vi "mux10_1(x6)_encode.vi"(8 "error in (no error)":errorcluster, 10 "mux10_1(x6)_encode":T1(ring), 11 "Mem_mapping in":u16[](array[numeric])) -> (0 "error out":errorcluster, 3 "MemMapping Out":u16[](array[numeric]))   [LabVIEW 2018, in "MB Relay.lvlib"]
uses:
  MB Relay.lvlib
panel:
  out "mux1_10(x6)":u16[](array[numeric])
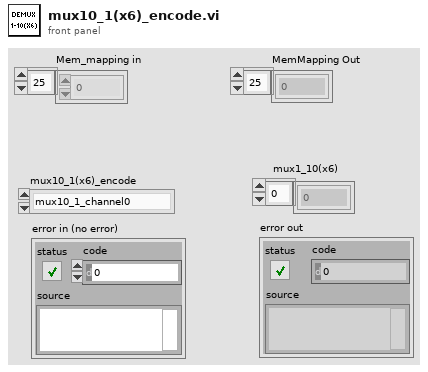
[diagram p1: front panel]
types:
  T1 = enum16{"mux10_1_channel0", "mux10_1_channel1", "mux10_1_channel2", "mux10_1_channel3", "mux10_1_channel4", "mux10_1_channel5", "mux10_1_channel6", "mux10_1_channel7", "mux10_1_channel8", "mux10_1_channel9", "mux10_1_channel10"}
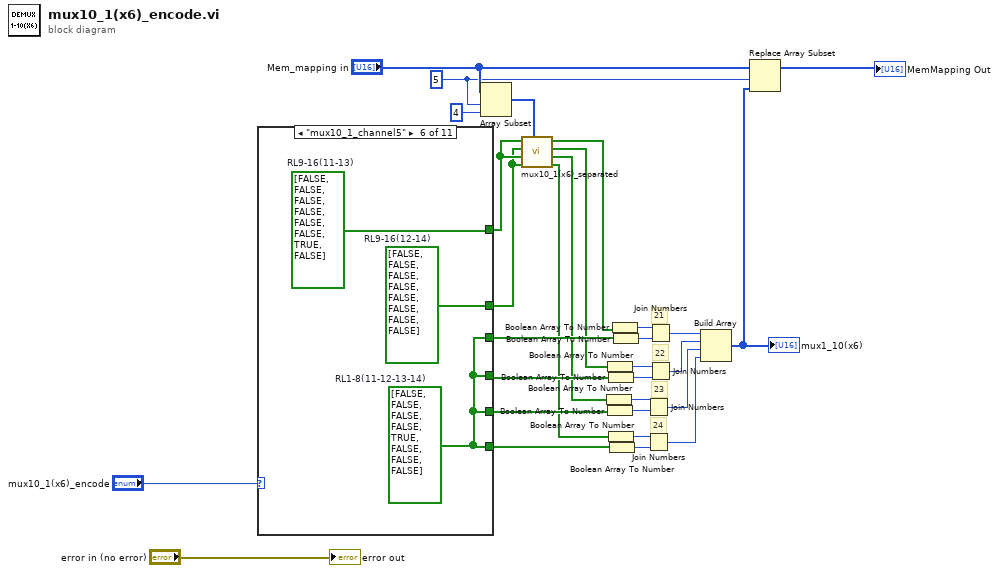
[diagram p0: block diagram]
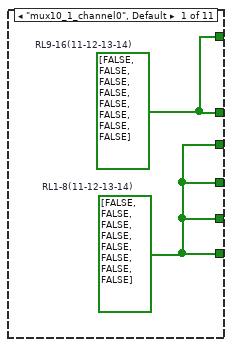
[diagram p2: hidden frame]
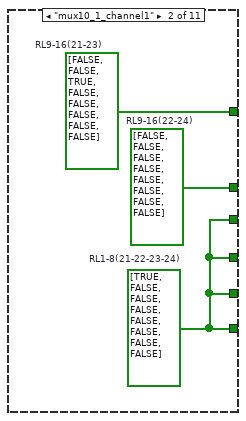
[diagram p3: hidden frame]
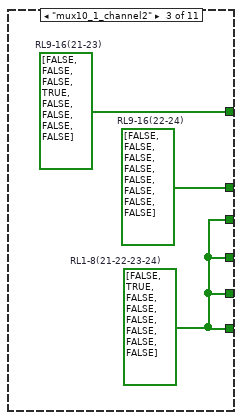
[diagram p4: hidden frame]
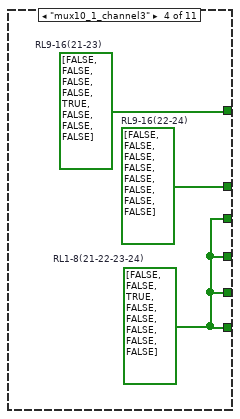
[diagram p5: hidden frame]
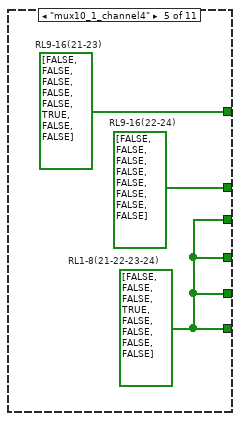
[diagram p6: hidden frame]
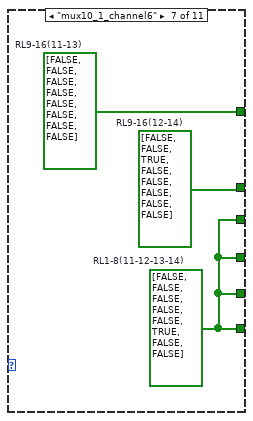
[diagram p7: hidden frame]
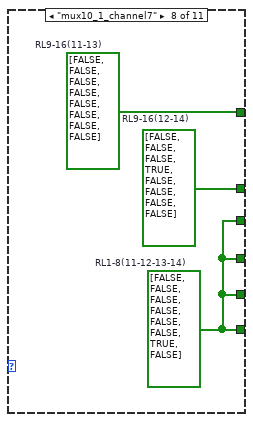
[diagram p8: hidden frame]
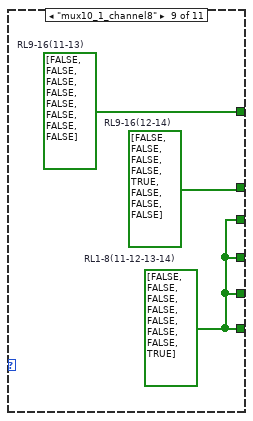
[diagram p9: hidden frame]
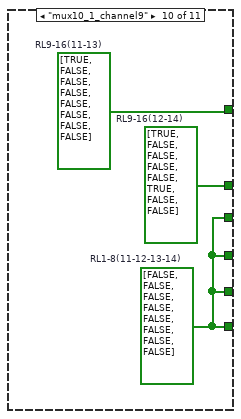
[diagram p10: hidden frame]
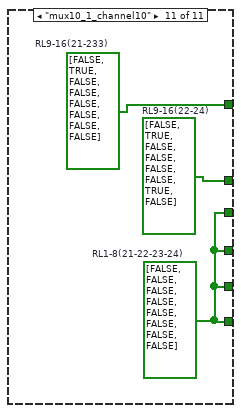
[diagram p11: hidden frame]
diagram:
  w8 = 5 ("index")
  # "24"
  # "23"
  # "22"
  # "21"
  n1 = case shown="\"mux10_1_channel5\"" "mux10_1(x6)_encode" {
    tunnel: [w32 w35 w38 w41 w44 w47 w50 w53 w56 w59 w62] -> w17
    tunnel: [w32 w35 w38 w41 w44 w47 w50 w53 w56 w59 w62] -> w18
    tunnel: [w32 w35 w38 w41 w44 w47 w50 w53 w56 w59 w62] -> w16
    tunnel: [w32 w35 w38 w41 w44 w47 w50 w53 w56 w59 w62] -> w21
    tunnel: [w31 w34 w37 w40 w43 w46 w49 w52 w55 w58 w61] -> w6
    tunnel: [w31 w33 w36 w39 w42 w45 w48 w51 w54 w57 w60] -> w5
    frame "mux10_1_channel0", Default {
      w31 = bool[] [FALSE, FALSE, FALSE, FALSE, FALSE, FALSE, FALSE, FALSE]  # RL9-16(11-12-13-14)
      w32 = bool[] [FALSE, FALSE, FALSE, FALSE, FALSE, FALSE, FALSE, FALSE]  # RL1-8(11-12-13-14)
    }
    frame "mux10_1_channel1" {
      w33 = bool[] [FALSE, FALSE, FALSE, FALSE, FALSE, FALSE, FALSE, FALSE]  # RL9-16(22-24)
      w34 = bool[] [FALSE, FALSE, TRUE, FALSE, FALSE, FALSE, FALSE, FALSE]  # RL9-16(21-23)
      w35 = bool[] [TRUE, FALSE, FALSE, FALSE, FALSE, FALSE, FALSE, FALSE]  # RL1-8(21-22-23-24)
    }
    frame "mux10_1_channel2" {
      w36 = bool[] [FALSE, FALSE, FALSE, FALSE, FALSE, FALSE, FALSE, FALSE]  # RL9-16(22-24)
      w37 = bool[] [FALSE, FALSE, FALSE, TRUE, FALSE, FALSE, FALSE, FALSE]  # RL9-16(21-23)
      w38 = bool[] [FALSE, TRUE, FALSE, FALSE, FALSE, FALSE, FALSE, FALSE]  # RL1-8(21-22-23-24)
    }
    frame "mux10_1_channel3" {
      w39 = bool[] [FALSE, FALSE, FALSE, FALSE, FALSE, FALSE, FALSE, FALSE]  # RL9-16(22-24)
      w40 = bool[] [FALSE, FALSE, FALSE, FALSE, TRUE, FALSE, FALSE, FALSE]  # RL9-16(21-23)
      w41 = bool[] [FALSE, FALSE, TRUE, FALSE, FALSE, FALSE, FALSE, FALSE]  # RL1-8(21-22-23-24)
    }
    frame "mux10_1_channel4" {
      w42 = bool[] [FALSE, FALSE, FALSE, FALSE, FALSE, FALSE, FALSE, FALSE]  # RL9-16(22-24)
      w43 = bool[] [FALSE, FALSE, FALSE, FALSE, FALSE, TRUE, FALSE, FALSE]  # RL9-16(21-23)
      w44 = bool[] [FALSE, FALSE, FALSE, TRUE, FALSE, FALSE, FALSE, FALSE]  # RL1-8(21-22-23-24)
    }
    frame "mux10_1_channel5" {
      w45 = bool[] [FALSE, FALSE, FALSE, FALSE, FALSE, FALSE, FALSE, FALSE]  # RL9-16(12-14)
      w46 = bool[] [FALSE, FALSE, FALSE, FALSE, FALSE, FALSE, TRUE, FALSE]  # RL9-16(11-13)
      w47 = bool[] [FALSE, FALSE, FALSE, FALSE, TRUE, FALSE, FALSE, FALSE]  # RL1-8(11-12-13-14)
    }
    frame "mux10_1_channel6" {
      w48 = bool[] [FALSE, FALSE, TRUE, FALSE, FALSE, FALSE, FALSE, FALSE]  # RL9-16(12-14)
      w49 = bool[] [FALSE, FALSE, FALSE, FALSE, FALSE, FALSE, FALSE, FALSE]  # RL9-16(11-13)
      w50 = bool[] [FALSE, FALSE, FALSE, FALSE, FALSE, TRUE, FALSE, FALSE]  # RL1-8(11-12-13-14)
    }
    frame "mux10_1_channel7" {
      w51 = bool[] [FALSE, FALSE, FALSE, TRUE, FALSE, FALSE, FALSE, FALSE]  # RL9-16(12-14)
      w52 = bool[] [FALSE, FALSE, FALSE, FALSE, FALSE, FALSE, FALSE, FALSE]  # RL9-16(11-13)
      w53 = bool[] [FALSE, FALSE, FALSE, FALSE, FALSE, FALSE, TRUE, FALSE]  # RL1-8(11-12-13-14)
    }
    frame "mux10_1_channel8" {
      w54 = bool[] [FALSE, FALSE, FALSE, FALSE, TRUE, FALSE, FALSE, FALSE]  # RL9-16(12-14)
      w55 = bool[] [FALSE, FALSE, FALSE, FALSE, FALSE, FALSE, FALSE, FALSE]  # RL9-16(11-13)
      w56 = bool[] [FALSE, FALSE, FALSE, FALSE, FALSE, FALSE, FALSE, TRUE]  # RL1-8(11-12-13-14)
    }
    frame "mux10_1_channel9" {
      w57 = bool[] [TRUE, FALSE, FALSE, FALSE, FALSE, TRUE, FALSE, FALSE]  # RL9-16(12-14)
      w58 = bool[] [TRUE, FALSE, FALSE, FALSE, FALSE, FALSE, FALSE, FALSE]  # RL9-16(11-13)
      w59 = bool[] [FALSE, FALSE, FALSE, FALSE, FALSE, FALSE, FALSE, FALSE]  # RL1-8(11-12-13-14)
    }
    frame "mux10_1_channel10" {
      w60 = bool[] [FALSE, TRUE, FALSE, FALSE, FALSE, FALSE, TRUE, FALSE]  # RL9-16(22-24)
      w61 = bool[] [FALSE, TRUE, FALSE, FALSE, FALSE, FALSE, FALSE, FALSE]  # RL9-16(21-233)
      w62 = bool[] [FALSE, FALSE, FALSE, FALSE, FALSE, FALSE, FALSE, FALSE]  # RL1-8(21-22-23-24)
    }
  }
  n2 = Array Subset(array="Mem_mapping in", index=w8, length=4) -> (w7:u16[])
  n3 = call "mux10_1(x6)_separated.vi"("Mem_mapping in"=w7, "Boolean array 24"=w5, "Boolean array 23"=w6, "Boolean array 22"=w5, "Boolean array 21"=w6) -> ("output array 24"=w4:bool[], "output array 23"=w3:bool[], "output array 22"=w2:bool[], "output array 21"=w1:bool[])  [unwired: 3 in]
  n4 = Boolean Array To Number(Boolean array=w3) -> (number=w14:u8)
  n5 = Boolean Array To Number(Boolean array=w2) -> (number=w15:u8)
  n6 = Boolean Array To Number(Boolean array=w18) -> (number=w13:u8)
  n7 = Boolean Array To Number(Boolean array=w16) -> (number=w19:u8)
  n8 = Boolean Array To Number(Boolean array=w4) -> (number=w12:u8)
  n9 = Boolean Array To Number(Boolean array=w17) -> (number=w11:u8)
  n10 = Boolean Array To Number(Boolean array=w1) -> (number=w22:u8)
  n11 = Boolean Array To Number(Boolean array=w21) -> (number=w20:u8)
  n12 = Join Numbers(hi=w14, lo=w13) -> ((hi.lo)=w27:u16)
  n13 = Join Numbers(hi=w12, lo=w11) -> ((hi.lo)=w28:u16)
  n14 = Join Numbers(hi=w22, lo=w20) -> ((hi.lo)=w25:u16)
  n15 = Join Numbers(hi=w15, lo=w19) -> ((hi.lo)=w26:u16)
  n16 = Build Array(w25, w26, w27, w28) -> (w10:u16[])
  "mux1_10(x6)" <- w10
  n17 = Replace Array Subset(array="Mem_mapping in", new element=w10, index=w8) -> (→"MemMapping Out":u16[])
  "error out" <- "error in (no error)"
